vi "DIOToString.vi"(8 "error in (no error)":errorcluster, 11 "DIO":T1) -> (0 "error out":errorcluster, 3 "DIO String":string)   [LabVIEW 2012]
uses:
  2013-Competition_Dash/DIOOutput.ctl
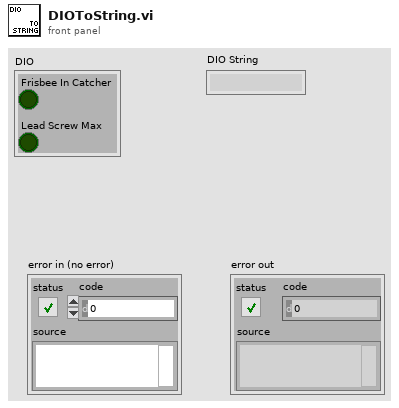
[diagram p1: front panel]
types:
  T1 = typedef "DIOOutput.ctl" = cluster{"Frisbee In Catcher":bool, "Lead Screw Max":bool}
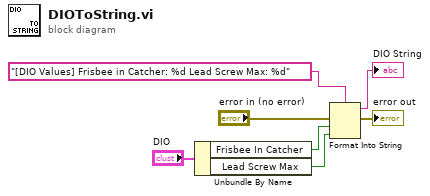
[diagram p0: block diagram]
diagram:
  n1 = Unbundle By Name("DIO") -> ("Frisbee In Catcher"=w7:bool, "Lead Screw Max"=w6:bool)
  n2 = Format Into String(format string="[DIO Values] Frisbee in Catcher: %d Lead Screw Max: %d", error in="error in (no error)", w7, w6) -> (resulting string=→"DIO String":string, error out=→"error out":errorcluster)  [unwired: 1 in]
